vi "LINC Read Telemetry.vi"(5 "start field (-1)":i32=-1, 6 "options":T1, 7 "mode (single)":enum16{"single", "packet", "all"}(ring), 8 "error in (no error)":errorcluster, 9 "item name":string, 10 "packet name":string, 11 "LINC session":refnum<class "LINC.lvclass">) -> (0 "error out":errorcluster, 1 "item values":string[](array[string]), 2 "item names":string[](array[string]), 3 "dup LINC session":refnum<class "LINC.lvclass">, 4 "flattened data":string)   [LabVIEW 2018, in "STEPkgDriver_LINC.lvlib" / "LINC.lvclass"]
uses:
  LINC.lvclass
  STEPkgDriver_LINC.lvlib
  LINC Global Mode.ctl
  LINC Global Config Mode.ctl
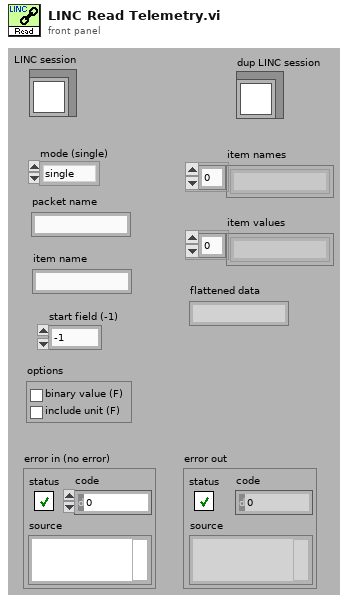
[diagram p1: front panel]
types:
  T1 = cluster{"binary value (F)":bool, "include unit (F)":bool}
  T2 = typedef "STEPkgDriver_LINC.lvlib/LINC Global Mode.ctl" = enum16{"INIT", "CLEAR", "ADD_PKT_HDR", "ADD_PKT", "GET_PKT_NAMES", "GET_PKT_DESC", "GET_PKT_HDR", "GET_PKT", "SET_PKT", "SET_DATA", "SIM_EN", "SIM_DS"}
  T3 = typedef "STEPkgDriver_LINC.lvlib/LINC Global Config Mode.ctl" = enum16{"INIT", "CLEAR", "SET_CMD_CB", "SET_TLM_CB", "SET_CMD_FIELDS", "SET_TLM_FIELDS", "SET_ID", "GET_CONFIG"}
  T4 = typedef "STEPkgDriver_LINC.lvlib/LINC Format Prototype.ctl" = cluster{"type":string, "bit offset":i32, "bit size":i32, "format":string, "unit":string, "description":string, "state values":i64[], "states":string[], "max":string, "min":string, "default":string, "array":bool, "bit element size":i32, "poly bound":dbl[], "poly scale":cluster{"coefficients":dbl[]}[], "labview size":i32, "simulate":bool, "ID":bool, "required":bool}
  T5 = typedef "STEPkgDriver_LINC.lvlib/LINC Config.ctl" = cluster{"cmd callback":refnum<vi>, "tlm callback":refnum<vi>, "cmd ID bitoffset":i32, "cmd ID bitsize":i32, "cmd IDs":i32[], "tlm ID bitoffset":i32, "tlm ID bitsize":i32, "tlm IDs":i32[], "cmd header fields":i32, "tlm header fields":i32, "tlm header size":i32}
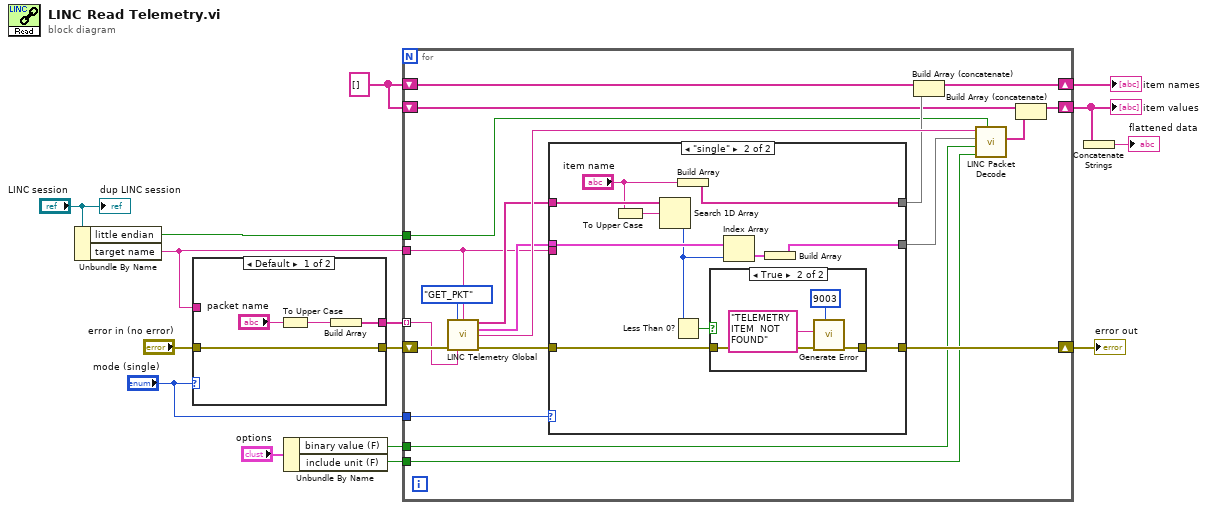
[diagram p0: block diagram]
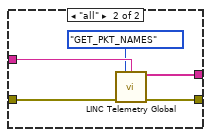
[diagram p2: hidden frame]
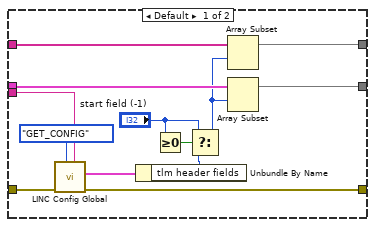
[diagram p3: hidden frame]
diagram:
  w8 = string[] []
  n1 = Unbundle By Name("LINC session") -> ("little endian"=w1:bool, "target name"=w11:string)
  n2 = case shown="Default" "mode (single)" {
    tunnel: "error in (no error)" -> [w19 w24]
    tunnel: [w19 w23] -> w12
    tunnel: w11 -> [_ w22]
    tunnel: [w18 w21] -> w10
    frame Default {
      n3 = To Upper Case(1:"packet name") -> (0:w16:string)
      n4 = Build Array(w16) -> (w18:string[])
    }
    frame "all" {
      n5 = call "LINC Telemetry Global.vi"("mode"=LINC_Global_Mode."GET_PKT_NAMES", "target name"=w22, "error in (no error)"=w24) -> ("values out"=w21:string[], "error out"=w23:errorcluster)  [unwired: 8 in, 3 out]
    }
  }
  n6 = Unbundle By Name("options") -> ("binary value (F)"=w3:bool, "include unit (F)"=w2:bool)
  n7 = for {
    tunnel: w11 -> [w25]
    shift-right: [w32] -> w14
    shift-left: w12 -> [w43]
    tunnel: w10 -> [w27] mode=indexing
    tunnel: "mode (single)" -> [w40]
    shift-right: [w31] -> w6
    shift-left: w8 -> [w34]
    shift-right: [w35] -> w7
    shift-left: w8 -> [w37]
    tunnel: w3 -> [w29]
    tunnel: w2 -> [w28]
    tunnel: w1 -> [w26]
    n8 = call "LINC Telemetry Global.vi"("mode"=LINC_Global_Mode."GET_PKT", "target name"=w25, "error in (no error)"=w43, "packet name"=w27) -> ("values out"=w42:string[], "item formats out"=w41:T4[], "data out"=w44:string, "error out"=w38:errorcluster)  [unwired: 7 in, 1 out]
    n9 = case shown="\"single\"" w40 {
      tunnel: w42 -> [w57 w65]
      tunnel: w41 -> [w55 w62]
      tunnel: [w56 w64] -> w36
      tunnel: [w54 w59] -> w39
      tunnel: w38 -> [w53 w67]
      tunnel: [w52 w66] -> w32
      tunnel: w25 -> [w51 _]
      frame Default {
        n10 = call "LINC Config Global.vi"("target name"=w51, "mode"=LINC_Global_Config_Mode."GET_CONFIG", "error in (no error)"=w53) -> ("error out"=w52:errorcluster, "config out"=w49:T5)  [unwired: 7 in]
        n11 = Unbundle By Name(w49) -> ("tlm header fields"=w46:i32)
        n12 = Greater Or Equal To 0?(x="start field (-1)") -> (x >= 0?=w48:bool)
        n13 = Select(t="start field (-1)", s=w48, f=w46) -> (s? t:f=w45:i32)
        n14 = Array Subset(array=w57, index=w45) -> (w56:string[])  [unwired: 1 in]
        n15 = Array Subset(array=w55, index=w45) -> (w54:T4[])  [unwired: 1 in]
      }
      frame "single" {
        n16 = To Upper Case(1:"item name") -> (0:w58:string)
        n17 = Search 1D Array(1D array=w65, element=w58) -> (index of element=w61:i32)  [unwired: 1 in]
        n18 = Less Than 0?(x=w61) -> (x < 0?=w68:bool)
        n19 = Build Array("item name") -> (w64:string[])
        n20 = case shown="True" w68 {
          tunnel: w67 -> [w69 w73]
          tunnel: [w69 w72] -> w66
          frame False {
          }
          frame True {
            n21 = call "Generate Error.vi"("error code (-1301)"=9003, "error in"=w73, "description"="TELEMETRY ITEM  NOT FOUND") -> ("error out"=w72:errorcluster)  [unwired: 8 in]
          }
        }
        n22 = Index Array(array=w62, index=w61) -> (element=w60:T4)
        n23 = Build Array(w60) -> (w59:T4[])
      }
    }
    n24 = Build Array (concatenate)(w37, w36) -> (w35:string[])
    n25 = call "LINC Packet Decode.vi"("little endian"=w26, "include unit (F)"=w28, "binary value (F)"=w29, "item formats"=w39, "data in"=w44) -> ("decoded items"=w33:string[])  [unwired: 6 in]
    n26 = Build Array (concatenate)(w34, w33) -> (w31:string[])
  }
  "error out" <- w14
  "item names" <- w7
  "item values" <- w6
  n27 = Concatenate Strings(w6) -> (→"flattened data":string)
  "dup LINC session" <- "LINC session"
